vi "All-Indentify-To-Sort.vi"(8 "Error In":errorcluster, 11 "輸出顏色-位置":T1(array[cluster])) -> (0 "Error Out":errorcluster, 1 "輸出移動值2":dbl[](array[numeric]), 2 "執行放球?":bool, 3 "輸出移動值":dbl[](array[numeric]), 5 "執行補值、校正?":bool)   [LabVIEW 2019]
uses:
  Variable/Indentify-Consequent.vi
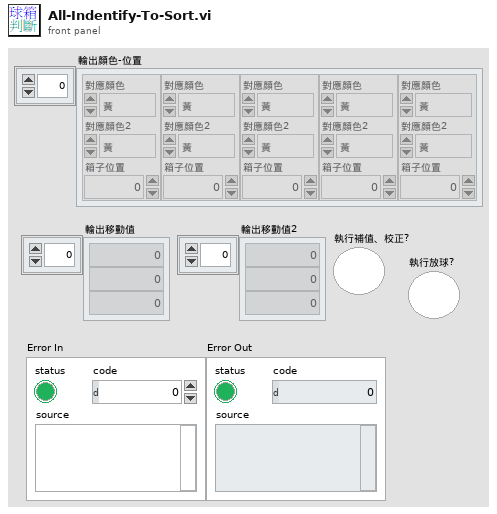
[diagram p1: front panel]
types:
  T1 = cluster{"對應顏色":enum16{"黃", "紅", "綠", "藍", "黑", "無"}, "對應顏色2":enum16{"黃", "紅", "綠", "藍", "黑", "無"}, "箱子位置":i32}[]
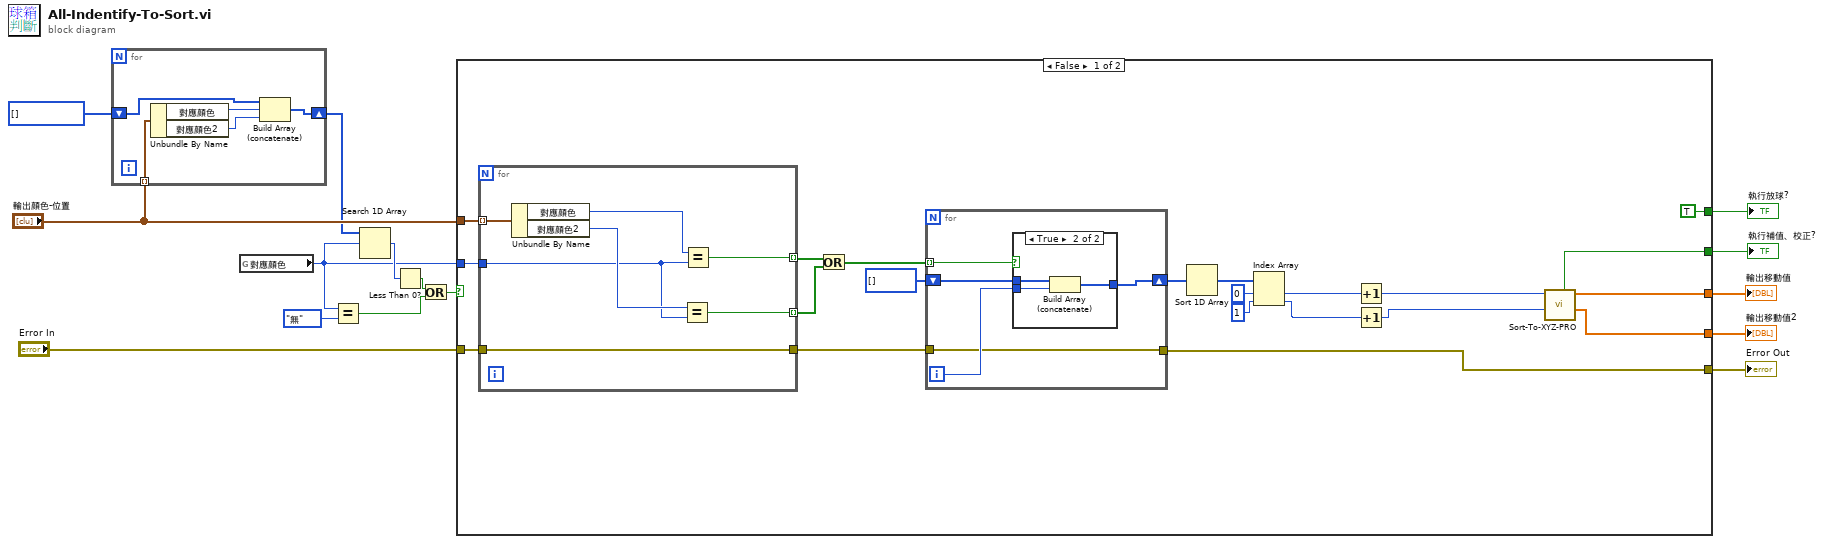
[diagram p0: block diagram]
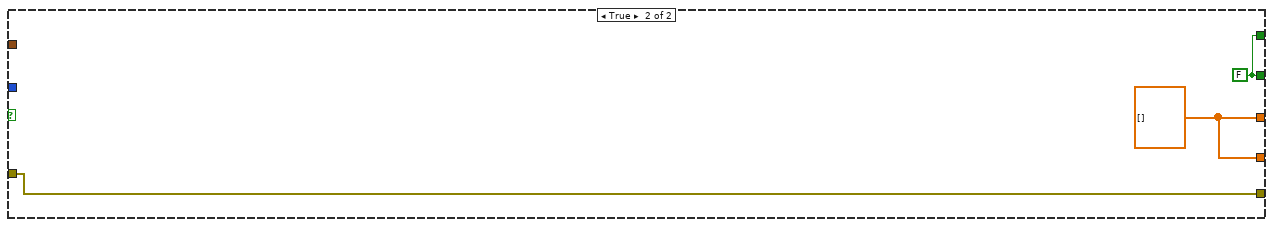
[diagram p3: hidden frame]
diagram:
  w3 = enum16{"黃", "紅", "綠", "藍", "黑", "無"}[] [] items=["黃", "紅", "綠", "藍", "黑", "無"]
  n1 = for {
    tunnel: "輸出顏色-位置" -> [w20] mode=indexing
    shift-right: [w17] -> w2
    shift-left: w3 -> [w16]
    n2 = Unbundle By Name(w20) -> ("對應顏色"=w19:enum16{"黃", "紅", "綠", "藍", "黑", "無"}, "對應顏色2"=w18:enum16{"黃", "紅", "綠", "藍", "黑", "無"})
    n3 = Build Array (concatenate)(w16, w19, w18) -> (w17:enum16{"黃", "紅", "綠", "藍", "黑", "無"}[])
  }
  n4 = global read "Indentify-Consequent.vi" "對應顏色"() -> (w1:enum16{"黃", "紅", "綠", "藍", "黑", "無"})
  n5 = Equal?(x=w1, y=enum16{"黃", "紅", "綠", "藍", "黑", "無"}."無") -> (x = y?=w7:bool)
  n6 = Search 1D Array(1D array=w2, element=w1) -> (index of element=w5:i32)  [unwired: 1 in]
  n7 = Less Than 0?(x=w5) -> (x < 0?=w6:bool)
  n8 = Or(x=w6, y=w7) -> (x .or. y?=w8:bool)
  n9 = case shown="False" w8 {
    tunnel: "輸出顏色-位置" -> [w31 _]
    tunnel: w1 -> [w30 _]
    tunnel: "Error In" -> [w29 w58]
    tunnel: [w27 w58] -> w14
    tunnel: [w24 w60] -> w13
    tunnel: [w23 w60] -> w12
    tunnel: [w22 w59] -> w11
    tunnel: [TRUE ("放球校正?") w59] -> w9
    frame False {
      n10 = for {
        tunnel: w31 -> [w57] mode=indexing
        tunnel: w30 -> [w54]
        tunnel: [w53] -> w36 mode=indexing
        tunnel: [w52] -> w35 mode=indexing
        tunnel: [w51] -> w28
        tunnel: w29 -> [w51]
        n11 = Unbundle By Name(w57) -> ("對應顏色"=w56:enum16{"黃", "紅", "綠", "藍", "黑", "無"}, "對應顏色2"=w55:enum16{"黃", "紅", "綠", "藍", "黑", "無"})
        n12 = Equal?(x=w55, y=w54) -> (x = y?=w53:bool)
        n13 = Equal?(x=w56, y=w54) -> (x = y?=w52:bool)
      }
      n14 = Or(x=w35, y=w36) -> (x .or. y?=w34:bool[])
      n15 = for {
        tunnel: w34 -> [w46] mode=indexing
        shift-right: [w44] -> w32
        shift-left: i32[] [] -> [w43]
        tunnel: [w42] -> w27
        tunnel: w28 -> [w42]
        i -> [w45]
        n16 = case shown="True" w46 {
          tunnel: w45 -> [_ w50]
          tunnel: [w47 w49] -> w44
          tunnel: w43 -> [w47 w48]
          frame False {
          }
          frame True {
            n17 = Build Array (concatenate)(w48, w50) -> (w49:i32[])
          }
        }
      }
      n18 = Sort 1D Array(array=w32) -> (sorted array=w41:i32[])
      n19 = Index Array(array=w41, index #1=0 ("index"), index #2=1 ("index")) -> (element #1=w37:i32, element #2=w38:i32)
      n20 = Increment(x=w37) -> (x+1=w26:i32)
      n21 = Increment(x=w38) -> (x+1=w25:i32)
      n22 = call "Sort-To-XYZ-PRO.vi"("位置 2"=w25, "位置"=w26) -> ("移動二"=w23:dbl[], "移動一"=w24:dbl[], "放球校正?"=w22:bool)  [unwired: 7 in]
    }
    frame True {
      w60 = dbl[] [] ("移動一")
      w59 = FALSE ("放球校正?")
    }
  }
  "輸出移動值" <- w13
  "輸出移動值2" <- w12
  "執行補值、校正?" <- w11
  "Error Out" <- w14
  "執行放球?" <- w9
